vi "Page_Advanced_Initialize.vi"(6 "ctl references":T1, 8 "error in (no error)":errorcluster, 11 "AB_InteropAssembly in":refnum<class "AB_InteropAssembly.lvclass">) -> (0 "error out":errorcluster, 3 "AB_InteropAssembly out":refnum<class "AB_InteropAssembly.lvclass">)   [LabVIEW 2020, in "AB_InteropAssembly.lvclass"]
uses:
  <vilib>/AppBuilder/AB_Classes/InteropAssembly/AB_InteropAssembly.lvclass
  <resource>/Framework/Providers/Builds/AppBuilder/AB_UI_Page_Advanced_References.ctl
  <resource>/Framework/Providers/Common/provcom_StringGlobals.vi
  <vilib>/AppBuilder/AB_Classes/Application/AB_Application.lvclass
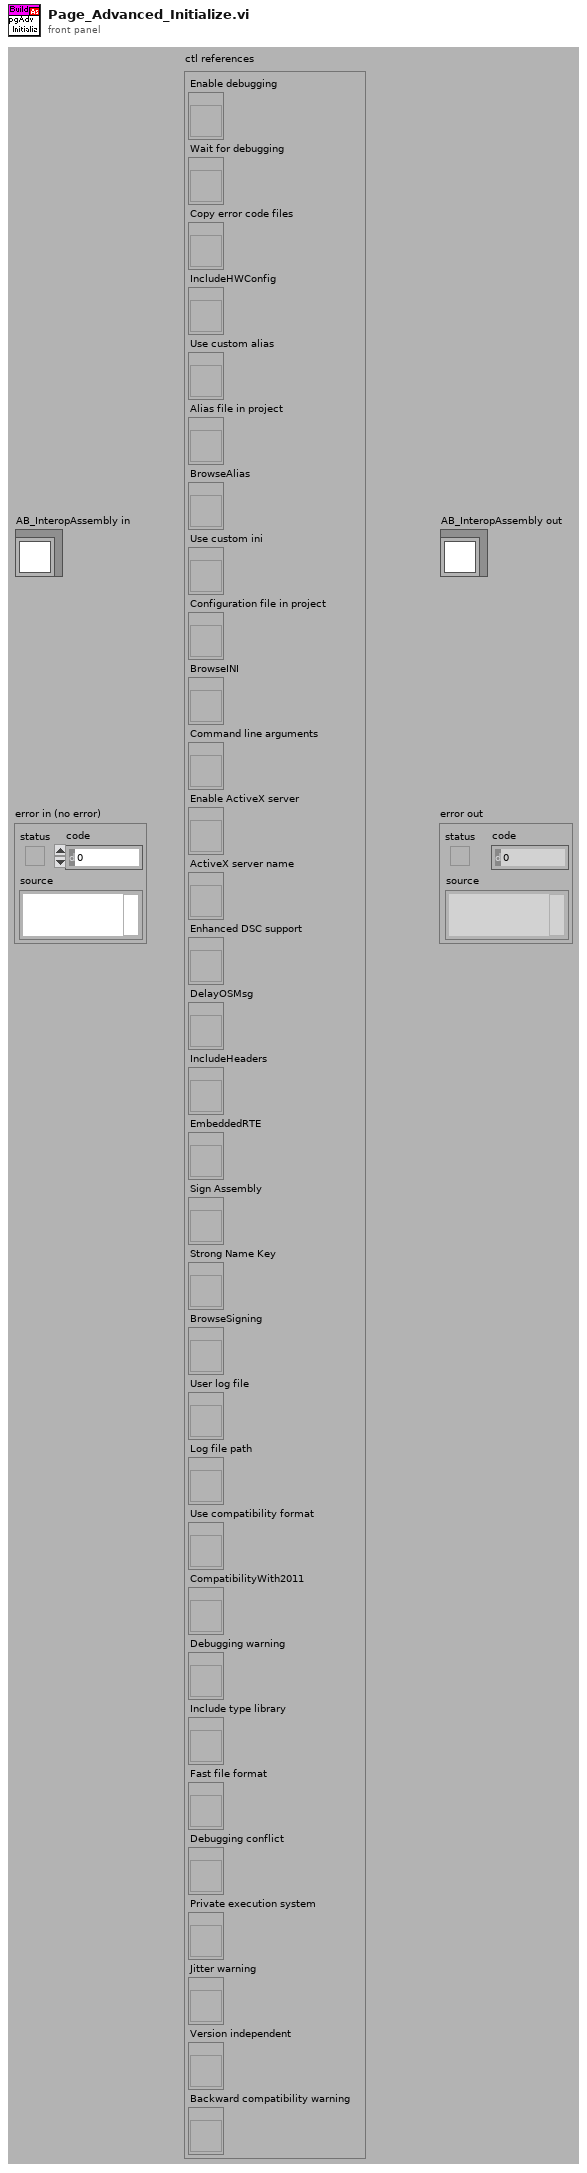
[diagram p1: front panel]
types:
  T1 = typedef "AB_UI_Page_Advanced_References.ctl" = cluster{"Enable debugging":refnum<vi>, "Wait for debugging":refnum<vi>, "Copy error code files":refnum<vi>, "IncludeHWConfig":refnum<vi>, "Use custom alias":refnum<vi>, "Alias file in project":refnum<vi>, "BrowseAlias":refnum<vi>, "Use custom ini":refnum<vi>, "Configuration file in project":refnum<vi>, "BrowseINI":refnum<vi>, "Command line arguments":refnum<vi>, "Enable ActiveX server":refnum<vi>, "ActiveX server name":refnum<vi>, "Enhanced DSC support":refnum<vi>, "DelayOSMsg":refnum<vi>, "IncludeHeaders":refnum<vi>, "EmbeddedRTE":refnum<vi>, "Sign Assembly":refnum<vi>, "Strong Name Key":refnum<vi>, "BrowseSigning":refnum<vi>, "User log file":refnum<vi>, "Log file path":refnum<vi>, "Use compatibility format":refnum<vi>, "CompatibilityWith2011":refnum<vi>, "Debugging warning":refnum<vi>, "Include type library":refnum<vi>, "Fast file format":refnum<vi>, "Debugging conflict":refnum<vi>, "Private execution system":refnum<vi>, "Jitter warning":refnum<vi>, "Version independent":refnum<vi>, "Backward compatibility warning":refnum<vi>}
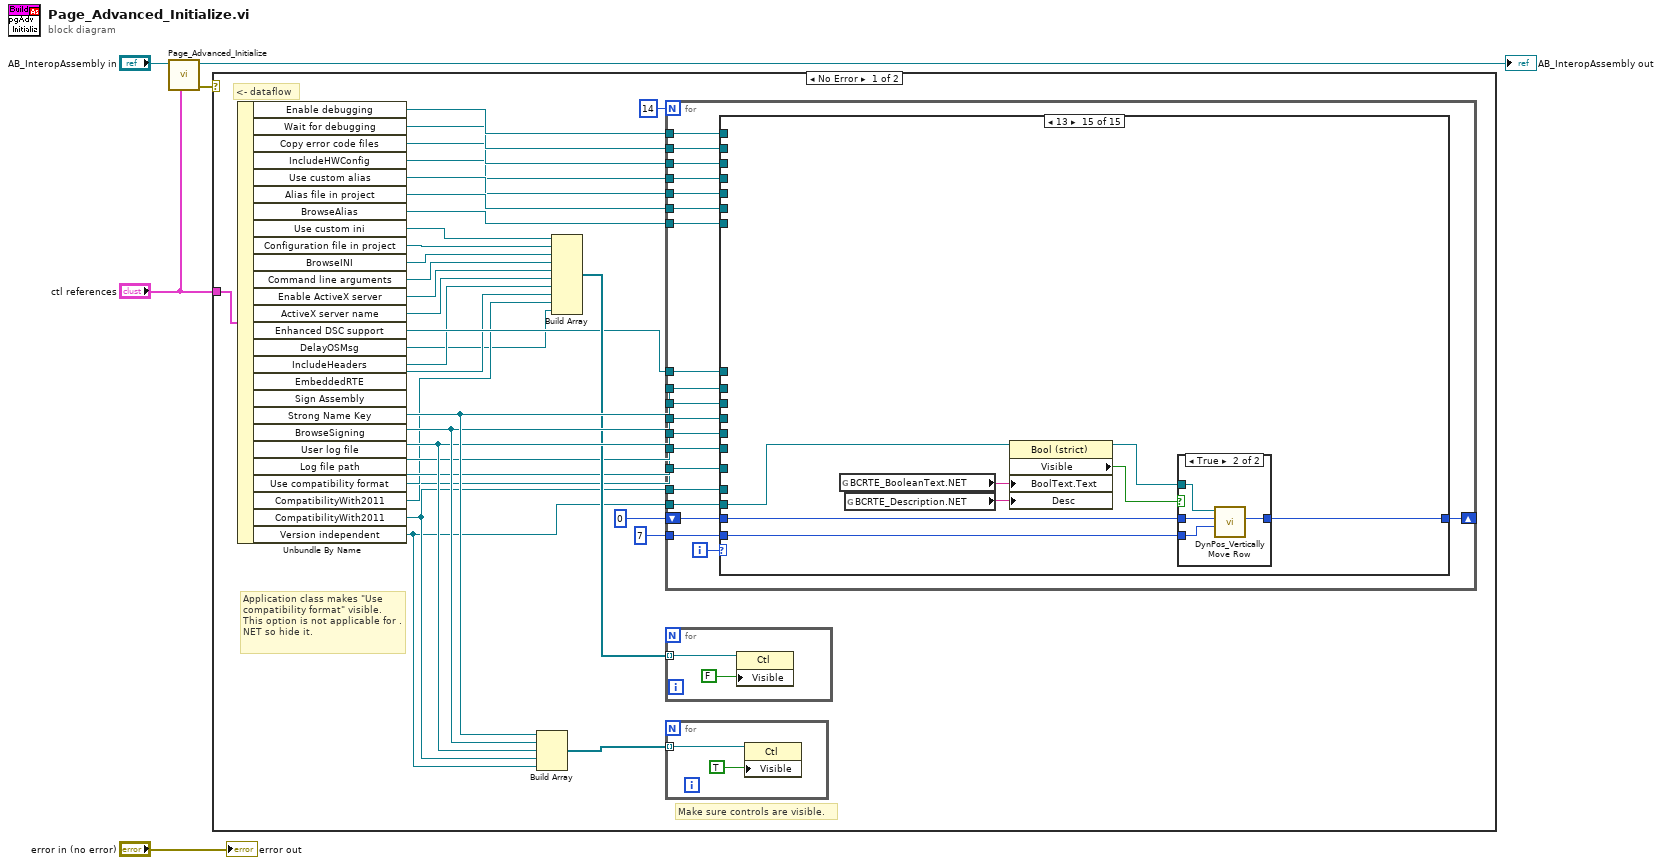
[diagram p0: block diagram]
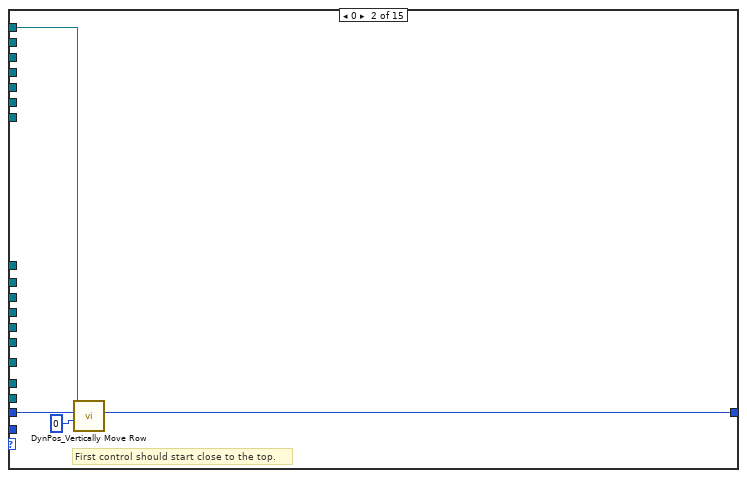
[diagram p3: hidden frame]
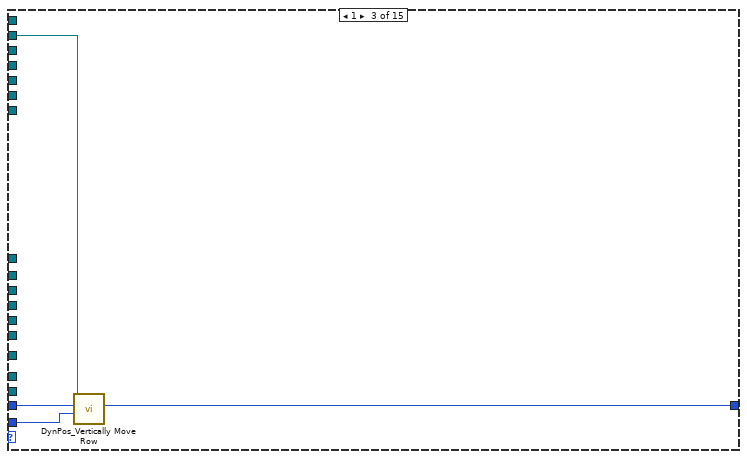
[diagram p4: hidden frame]
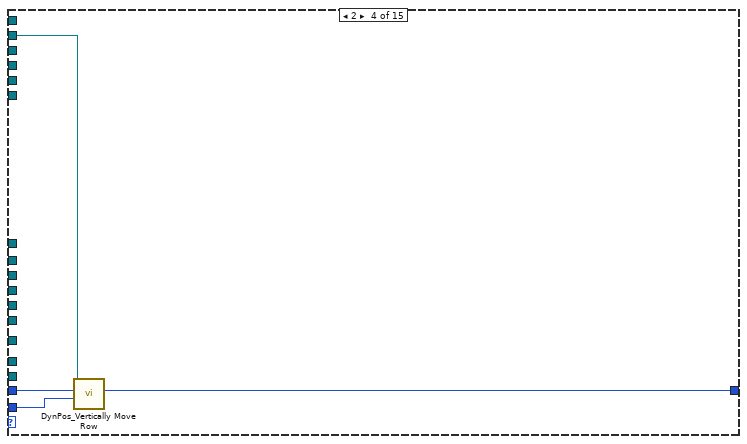
[diagram p5: hidden frame]
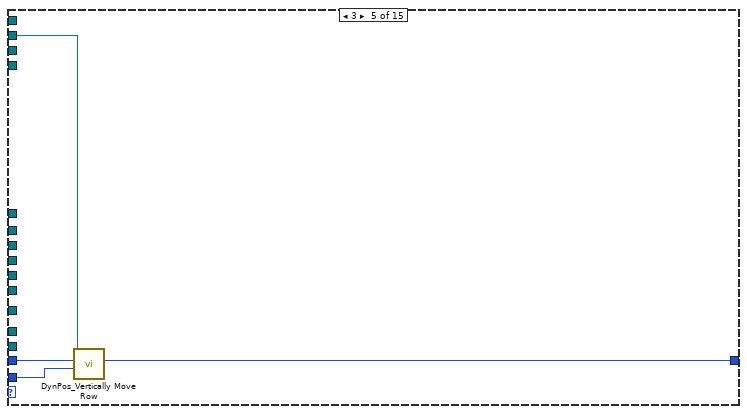
[diagram p6: hidden frame]
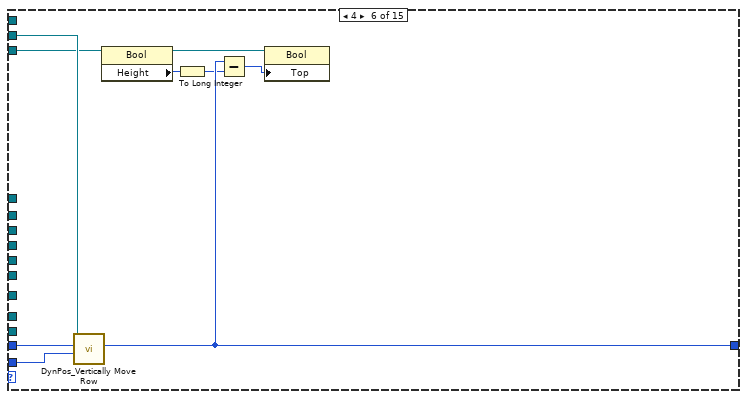
[diagram p7: hidden frame]
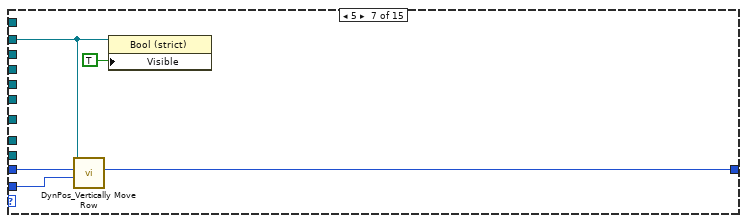
[diagram p8: hidden frame]
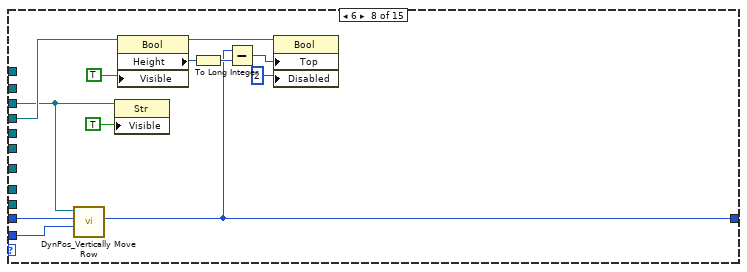
[diagram p9: hidden frame]
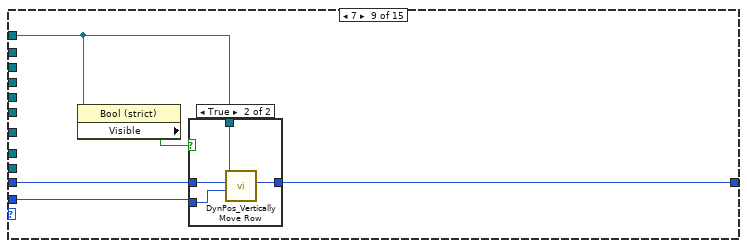
[diagram p10: hidden frame]
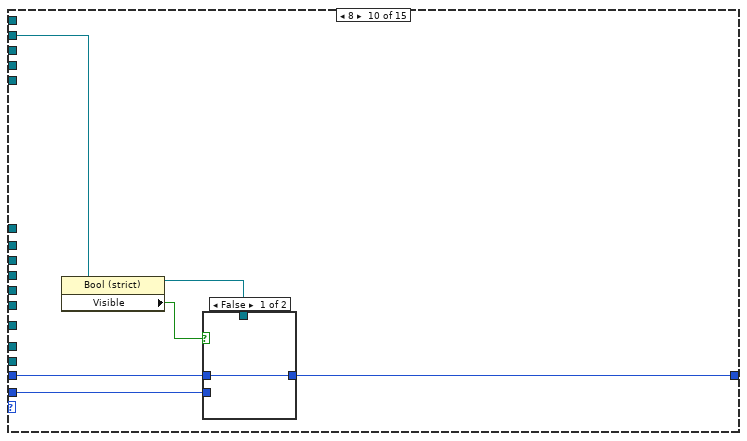
[diagram p12: hidden frame]
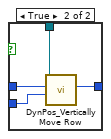
[diagram p13: hidden frame]
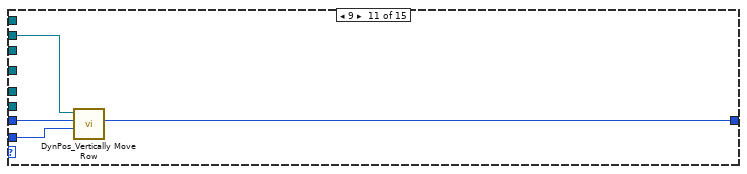
[diagram p14: hidden frame]
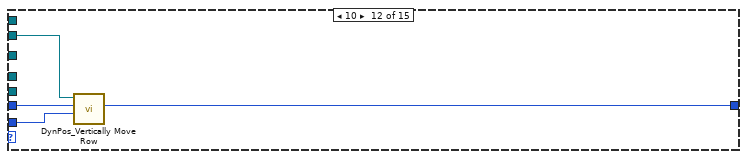
[diagram p15: hidden frame]
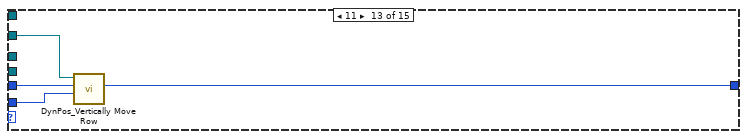
[diagram p16: hidden frame]
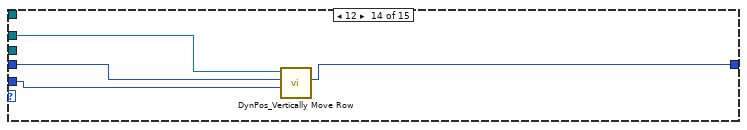
[diagram p17: hidden frame]
diagram:
  n1 = call-parent "Page_Advanced_Initialize.vi"("ctl references"="ctl references", "AB_Application in"="AB_InteropAssembly in") -> ("error out"=w1:errorcluster, "AB_Application out"=→"AB_InteropAssembly out":refnum<class "AB_InteropAssembly.lvclass">)  [unwired: 1 in, 7 out]
  n2 = case shown="No Error" w1 {
    tunnel: "ctl references" -> [w33 _]
    frame No Error {
      # "Application class makes \"Use compatibility format\" visible. This option is not applicable for .NET so hide it."
      # "<- dataflow"
      # "Make sure controls are visible."
      n3 = Unbundle By Name(w33) -> ("Enable debugging"=w26:refnum<vi>, "Wait for debugging"=w25:refnum<vi>, "Copy error code files"=w24:refnum<vi>, "IncludeHWConfig"=w11:refnum<vi>, "Use custom alias"=w17:refnum<vi>, "Alias file in project"=w23:refnum<vi>, "BrowseAlias"=w22:refnum<vi>, "Use custom ini"=w32:refnum<vi>, "Configuration file in project"=w31:refnum<vi>, "BrowseINI"=w27:refnum<vi>, "Command line arguments"=w30:refnum<vi>, "Enable ActiveX server"=w29:refnum<vi>, "ActiveX server name"=w28:refnum<vi>, "Enhanced DSC support"=w16:refnum<vi>, "DelayOSMsg"=w9:refnum<vi>, "IncludeHeaders"=w15:refnum<vi>, "EmbeddedRTE"=w14:refnum<vi>, "Sign Assembly"=w21:refnum<vi>, "Strong Name Key"=w20:refnum<vi>, "BrowseSigning"=w19:refnum<vi>, "User log file"=w13:refnum<vi>, "Log file path"=w12:refnum<vi>, "Use compatibility format"=w10:refnum<vi>, "CompatibilityWith2011"=w8:refnum<vi>, "CompatibilityWith2011"=w7:refnum<vi>, "Version independent"=w6:refnum<vi>)
      n4 = Build Array(w21, w20, w19, w7, w6) -> (w34:refnum<vi>[])
      n5 = Build Array(w32, w31, w27, w30, w29, w28, w15, w14, w10, w9) -> (w18:refnum<vi>[])
      n6 = for {
        N: 14 -> [_]
        shift-right: [w58] -> _
        shift-left: 0 ("Bottom of last control") -> [w60]
        tunnel: 7 ("Bottom of last control") -> [w59]
        tunnel: w26 -> [w57]
        tunnel: w25 -> [w56]
        tunnel: w24 -> [w55]
        tunnel: w17 -> [w54]
        tunnel: w23 -> [w53]
        tunnel: w22 -> [w52]
        tunnel: w21 -> [w51]
        tunnel: w20 -> [w50]
        tunnel: w19 -> [w49]
        tunnel: w16 -> [w48]
        tunnel: w13 -> [w47]
        tunnel: w12 -> [w46]
        tunnel: w11 -> [w45]
        tunnel: w8 -> [w44]
        tunnel: w7 -> [w43]
        tunnel: w6 -> [w42]
        i -> [w61]
        n7 = case shown="13" w61 {
          tunnel: w60 -> [w62 w66 w70 w74 w78 w87 w92 w104 w108 w118 w129 w133 w137 w141 w144]
          tunnel: w59 -> [_ _ w69 w73 w77 w86 w91 w103 w107 w117 w127 w131 w135 w140 w143]
          tunnel: [w62 w65 w68 w72 w76 w82 w90 w97 w106 w115 w128 w132 w136 w139 w142] -> w58
          tunnel: w57 -> [_ w63 _ _ _ _ _ _ _ _ _ _ _ _ _]
          tunnel: w56 -> [_ _ w67 _ _ _ _ _ _ _ _ _ _ _ _]
          tunnel: w55 -> [_ _ _ w71 _ _ _ _ _ _ _ _ _ _ _]
          tunnel: w54 -> [_ _ _ _ w75 _ _ _ _ _ _ _ _ _ _]
          tunnel: w53 -> [_ _ _ _ _ w80 _ _ _ _ _ _ _ _ _]
          tunnel: w52 -> [_ _ _ _ _ w79 _ _ _ _ _ _ _ _ _]
          tunnel: w51 -> [_ _ _ _ _ _ w89 _ _ _ _ _ _ _ _]
          tunnel: w50 -> [_ _ _ _ _ _ _ w93 _ _ _ _ _ _ _]
          tunnel: w49 -> [_ _ _ _ _ _ _ w98 _ _ _ _ _ _ _]
          tunnel: w48 -> [_ _ _ _ _ _ _ _ w105 _ _ _ _ _ _]
          tunnel: w47 -> [_ _ _ _ _ _ _ _ _ _ w126 _ _ _ _]
          tunnel: w46 -> [_ _ _ _ _ _ _ _ _ _ _ w130 _ _ _]
          tunnel: w45 -> [_ _ _ _ _ _ _ _ _ w119 _ _ _ _ _]
          tunnel: w44 -> [_ _ _ _ _ _ _ _ _ _ _ _ w134 _ _]
          tunnel: w43 -> [_ _ _ _ _ _ _ _ _ _ _ _ _ w138 _]
          tunnel: w42 -> [_ _ _ _ _ _ _ _ _ _ _ _ _ _ w145]
          frame Default {
          }
          frame 0 {
            # "First control should start close to the top."
            n8 = call <vilib>:"DynPos_Vertically Move Row.vi"("Pixel separation (6)"=0, "Bottom of last control"=w66, "Control"=w63) -> ("Bottom pixel"=w65:i32)  [unwired: 1 in, 7 out]
          }
          frame 1 {
            n9 = call <vilib>:"DynPos_Vertically Move Row.vi"("Pixel separation (6)"=w69, "Bottom of last control"=w70, "Control"=w67) -> ("Bottom pixel"=w68:i32)  [unwired: 1 in, 7 out]
          }
          frame 2 {
            n10 = call <vilib>:"DynPos_Vertically Move Row.vi"("Pixel separation (6)"=w73, "Bottom of last control"=w74, "Control"=w71) -> ("Bottom pixel"=w72:i32)  [unwired: 1 in, 7 out]
          }
          frame 3 {
            n11 = call <vilib>:"DynPos_Vertically Move Row.vi"("Pixel separation (6)"=w77, "Bottom of last control"=w78, "Control"=w75) -> ("Bottom pixel"=w76:i32)  [unwired: 1 in, 7 out]
          }
          frame 4 {
            n12 = call <vilib>:"DynPos_Vertically Move Row.vi"("Pixel separation (6)"=w86, "Bottom of last control"=w87, "Control"=w80) -> ("Bottom pixel"=w82:i32)  [unwired: 1 in, 7 out]
            n13 = property class="Bool"(reference=w79) -> (reference out=w85:refnum<vi>, "Height"=w84:u32)  [unwired: 1 in, 1 out]
            n14 = To Long Integer(number=w84) -> (32bit integer=w81:i32)
            n15 = Subtract(x=w82, y=w81) -> (x-y=w83:i32)
            n16 = property class="Bool"(reference=w85, "Top"=w83) -> ()  [unwired: 1 in, 2 out]
          }
          frame 5 {
            n17 = call <vilib>:"DynPos_Vertically Move Row.vi"("Pixel separation (6)"=w91, "Bottom of last control"=w92, "Control"=w89) -> ("Bottom pixel"=w90:i32)  [unwired: 1 in, 7 out]
            n18 = property class="Bool (strict)"(reference=w89, "Visible"=TRUE) -> ()  [unwired: 1 in, 2 out]
          }
          frame 6 {
            n19 = call <vilib>:"DynPos_Vertically Move Row.vi"("Pixel separation (6)"=w103, "Bottom of last control"=w104, "Control"=w93) -> ("Bottom pixel"=w97:i32)  [unwired: 1 in, 7 out]
            n20 = property class="Str"(reference=w93, "Visible"=TRUE) -> ()  [unwired: 1 in, 2 out]
            n21 = property class="Bool"(reference=w98, "Visible"=TRUE) -> (reference out=w102:refnum<vi>, "Height"=w101:u32)  [unwired: 1 in, 1 out]
            n22 = To Long Integer(number=w101) -> (32bit integer=w99:i32)
            n23 = Subtract(x=w97, y=w99) -> (x-y=w100:i32)
            n24 = property class="Bool"(reference=w102, "Top"=w100, "Disabled"=u8 2) -> ()  [unwired: 1 in, 2 out]
          }
          frame 7 {
            n25 = property class="Bool (strict)"(reference=w105) -> ("Visible"=w109:bool)  [unwired: 1 in, 2 out]
            n26 = case shown="True" w109 {
              tunnel: w108 -> [w110 w114]
              tunnel: w107 -> [_ w113]
              tunnel: [w110 w112] -> w106
              tunnel: w105 -> [_ w111]
              frame False {
              }
              frame True {
                n27 = call <vilib>:"DynPos_Vertically Move Row.vi"("Pixel separation (6)"=w113, "Bottom of last control"=w114, "Control"=w111) -> ("Bottom pixel"=w112:i32)  [unwired: 1 in, 7 out]
              }
            }
          }
          frame 8 {
            n28 = property class="Bool (strict)"(reference=w119) -> (reference out=w116:refnum<vi>, "Visible"=w120:bool)  [unwired: 1 in, 1 out]
            n29 = case shown="False" w120 {
              tunnel: w118 -> [w121 w125]
              tunnel: w117 -> [_ w124]
              tunnel: [w121 w123] -> w115
              tunnel: w116 -> [_ w122]
              frame False {
              }
              frame True {
                n30 = call <vilib>:"DynPos_Vertically Move Row.vi"("Pixel separation (6)"=w124, "Bottom of last control"=w125, "Control"=w122) -> ("Bottom pixel"=w123:i32)  [unwired: 1 in, 7 out]
              }
            }
          }
          frame 9 {
            n31 = call <vilib>:"DynPos_Vertically Move Row.vi"("Pixel separation (6)"=w127, "Bottom of last control"=w129, "Control"=w126) -> ("Bottom pixel"=w128:i32)  [unwired: 1 in, 7 out]
          }
          frame 10 {
            n32 = call <vilib>:"DynPos_Vertically Move Row.vi"("Pixel separation (6)"=w131, "Bottom of last control"=w133, "Control"=w130) -> ("Bottom pixel"=w132:i32)  [unwired: 1 in, 7 out]
          }
          frame 11 {
            n33 = call <vilib>:"DynPos_Vertically Move Row.vi"("Pixel separation (6)"=w135, "Bottom of last control"=w137, "Control"=w134) -> ("Bottom pixel"=w136:i32)  [unwired: 1 in, 7 out]
          }
          frame 12 {
            n34 = call <vilib>:"DynPos_Vertically Move Row.vi"("Pixel separation (6)"=w140, "Bottom of last control"=w141, "Control"=w138) -> ("Bottom pixel"=w139:i32)  [unwired: 1 in, 7 out]
          }
          frame 13 {
            n35 = global read "provcom_StringGlobals.vi" "BCRTE_BooleanText.NET"() -> (w147:string)
            n36 = global read "provcom_StringGlobals.vi" "BCRTE_Description.NET"() -> (w146:string)
            n37 = property class="Bool (strict)"(reference=w145, "BoolText.Text"=w147, "Desc"=w146) -> (reference out=w148:refnum<vi>, "Visible"=w149:bool)  [unwired: 1 in, 1 out]
            n38 = case shown="True" w149 {
              tunnel: w144 -> [w150 w154]
              tunnel: w143 -> [_ w153]
              tunnel: [w150 w152] -> w142
              tunnel: w148 -> [_ w151]
              frame False {
              }
              frame True {
                n39 = call <vilib>:"DynPos_Vertically Move Row.vi"("Pixel separation (6)"=w153, "Bottom of last control"=w154, "Control"=w151) -> ("Bottom pixel"=w152:i32)  [unwired: 1 in, 7 out]
              }
            }
          }
        }
      }
      n40 = for {
        tunnel: w18 -> [w40] mode=indexing
        n41 = property class="Ctl"(reference=w40, "Visible"=FALSE) -> ()  [unwired: 1 in, 2 out]
      }
      n42 = for {
        tunnel: w34 -> [w38] mode=indexing
        n43 = property class="Ctl"(reference=w38, "Visible"=TRUE) -> ()  [unwired: 1 in, 2 out]
      }
    }
    frame Error {
    }
  }
  "error out" <- "error in (no error)"
